vi "Script Custom Device.vi"(8 "error in":errorcluster, 10 "Parameter File Path":path, 11 "System Definition File Path In":path) -> (0 "error out":errorcluster, 1 "AIM ARINC 429 custom device out":T1 format="%.0x", 2 "System Definition Reference":refnum<k24>, 3 "System Definition File Path Out":path)   [LabVIEW 2020]
uses:
  Scripting/AIM/AIM ARINC 429 Scripting.lvlib
  niveristand-custom-device-testing-tools/VeriStandTestUtilities/VeriStandTestUtilities.lvlib
  Shared/Device Parameters.ctl
  <vilib>/NI VeriStand/Custom Device API/Custom Device Item Ref.ctl
  <vilib>/NI VeriStand/Custom Device API/Custom Device API.lvlib
  NationalInstruments.VeriStand.SystemDefinitionAPI
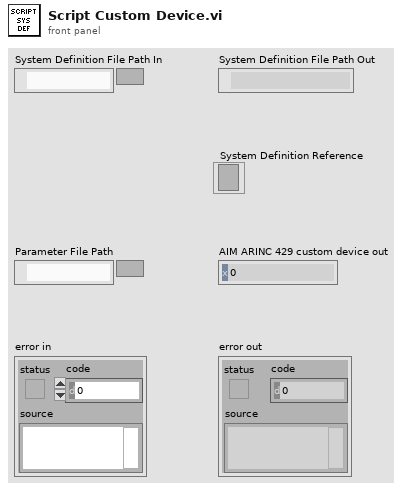
[diagram p1: front panel]
types:
  T1 = typedef "Custom Device API.lvlib/Custom Device Item Ref.ctl" = u64
  T2 = typedef "Device Parameters.ctl" = cluster{"pxi slot":u8}
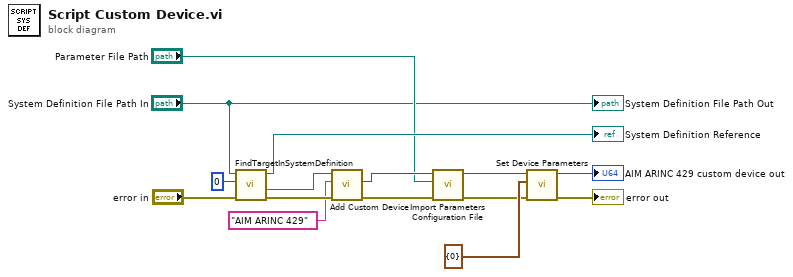
[diagram p0: block diagram]
diagram:
  n1 = call "FindTargetInSystemDefinition.vi"("error in"="error in", "target index"=0 ("index"), "system definition path"="System Definition File Path In") -> ("error out"=w14:errorcluster, "Target"=w13:refnum<k24>, "System Definition"=→"System Definition Reference":refnum<k24>)  [unwired: 5 in, 1 out]
  n2 = call "Add Custom Device.vi"("error in"=w14, "name"="AIM ARINC 429", "target in"=w13) -> ("error out"=w5:errorcluster, "AIM ARINC 429 custom device"=w4:T1)  [unwired: 6 in, 1 out]
  n3 = call "Import Parameters Configuration File.vi"("error in"=w5, "parameters configuration file path"="Parameter File Path", "AIM ARINC 429 custom device in"=w4) -> ("error out"=w7:errorcluster, "AIM ARINC 429 custom device out"=w6:T1)  [unwired: 7 in]
  n4 = call "Set Device Parameters.vi"("error in"=w7, "device parameters"=T2 {"pxi slot"=0}, "AIM ARINC 429 custom device in"=w6) -> ("error out"=→"error out":errorcluster, "AIM ARINC 429 custom device out"=→"AIM ARINC 429 custom device out":T1)  [unwired: 7 in]
  "System Definition File Path Out" <- "System Definition File Path In"
